vi "Write PV URL.vi"(8 "error in (no error)":errorcluster, 10 "PV URL":string, 11 "PVConnection in":refnum<class "PVConnection.lvclass">) -> (0 "error out":errorcluster, 3 "PVConnection out":refnum<class "PVConnection.lvclass">)   [LabVIEW 2012, in "CS++ProcessVariables.lvlib" / "PVConnection.lvclass"]
doc: "Write PV URL."
uses:
  PVConnection.lvclass
  PVConnection.lvclass/PVConnection.ctl
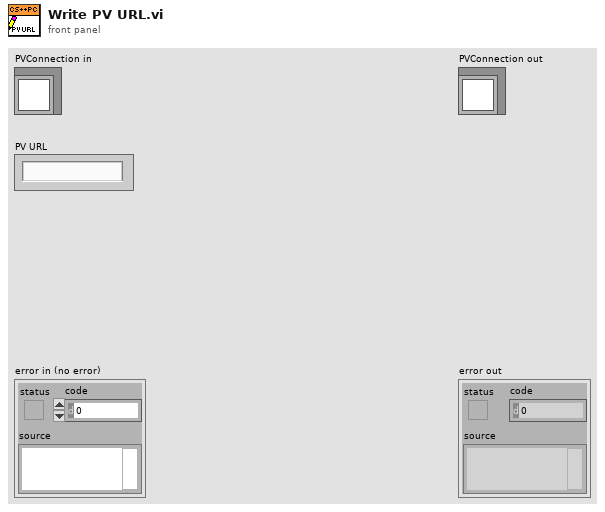
[diagram p1: front panel]
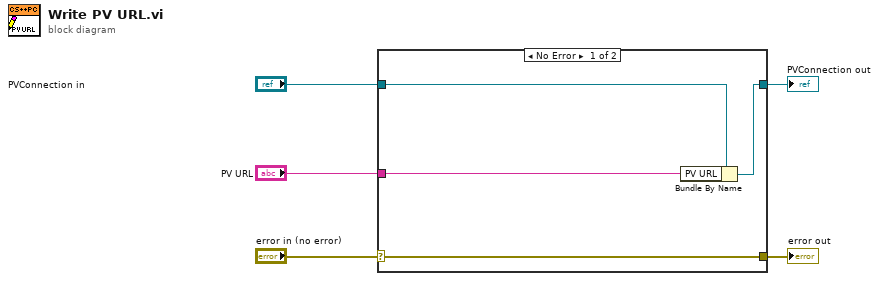
[diagram p0: block diagram]
diagram:
  n1 = case shown="No Error" "error in (no error)" {
    selector: "error in (no error)" -> [w9 w10]
    tunnel: [w9 w10] -> w4
    tunnel: [w7 w11] -> w2
    tunnel: "PVConnection in" -> [w8 w11]
    tunnel: "PV URL" -> [w6 _]
    frame No Error {
      n2 = Bundle By Name(cluster=w8, "PV URL"=w6) -> (w7:refnum<class "PVConnection.lvclass">)
    }
    frame Error {
    }
  }
  "error out" <- w4
  "PVConnection out" <- w2
